vi "BrewerisePlots.vi"(5 "graphRefnum":refnum<vi>, 7 "paletteRefnum":refnum<vi>, 8 "paletteNum":i32, 10 "Series":i32[](array[numeric]), 11 "Plot Legends":string[](array[string])) -> ()   [LabVIEW 2016]
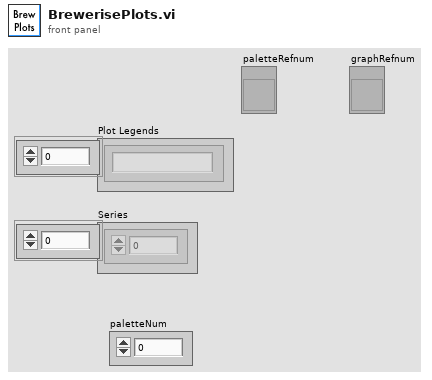
[diagram p1: front panel]
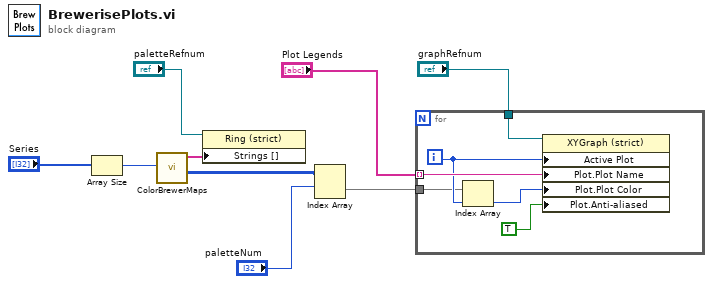
[diagram p0: block diagram]
diagram:
  n1 = Array Size(array="Series") -> (size(s)=w5:i32)
  n2 = call "ColorBrewerMaps.vi"("NSeries"=w5) -> ("allPalettes"=w6:u32[][], "availablePalettes"=w8:string[])  [unwired: 9 in]
  n3 = property on="Property Node" class="Ring (strict)"(reference="paletteRefnum", "Strings []"=w8) -> ()  [unwired: 1 in, 2 out]
  n4 = Index Array(array=w6, index (row)="paletteNum") -> (element=w9:u32[])  [unwired: 1 in]
  n5 = for {
    tunnel: "Plot Legends" -> [w15] mode=indexing
    tunnel: w9 -> [w13]
    tunnel: "graphRefnum" -> [w11]
    i -> [w14]
    n6 = Index Array(array=w13, index=w14) -> (element=w12:u32)
    n7 = property on="Property Node" class="XYGraph (strict)"(reference=w11, "Active Plot"=w14, "Plot.Plot Name"=w15, "Plot.Plot Color"=w12, "Plot.Anti-aliased"=TRUE) -> ()  [unwired: 1 in, 2 out]
  }
